vi "IBM4_Rate.vi"(8 "error in":errorcluster, 10 "Rate":i32=10000, 11 "COM resource in":refnum<visa-resource-name>="COM8") -> (0 "error out":errorcluster, 3 "COM resource out":refnum<visa-resource-name>="COM8")   [LabVIEW 2022 SP3, in "IBM4.lvlib"]
doc: "This VI interfaces with the IBM4 to perform a write operation where a Voltage is output on one of the analogue output pins of the IBM4.\n\nThe output channel must be 0 or 1, while the output value should be specified in Volts (thus, floating point)"
uses:
  <instrlib>/IBM4/IBM4.lvlib
panel:
  out "read buffer":string="Rate =  10000 SPS\r\n"
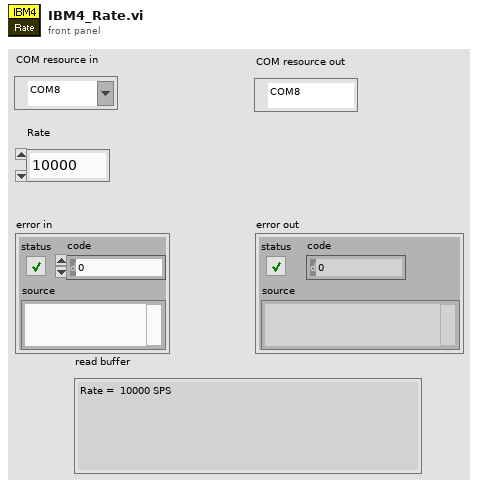
[diagram p1: front panel]
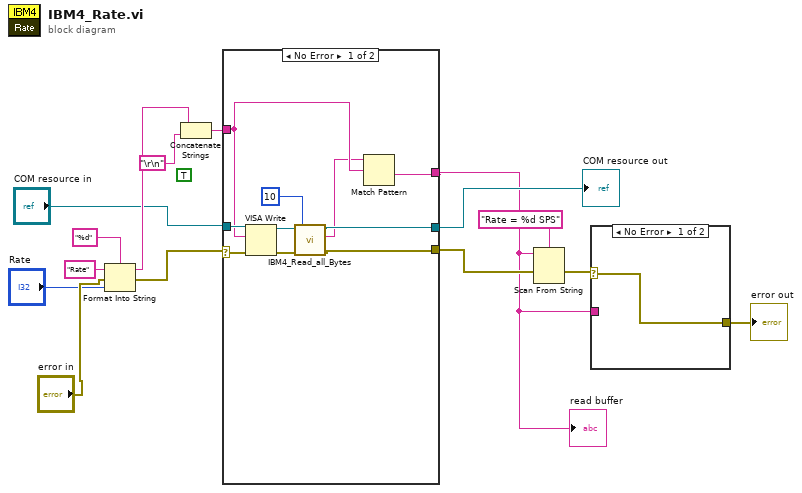
[diagram p0: block diagram]
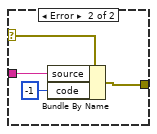
[diagram p2: hidden frame]
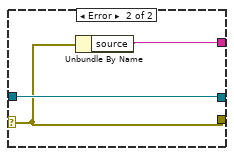
[diagram p3: hidden frame]
diagram:
  (unwired) TRUE ("Enable Termination\nChar (T)")
  n1 = Format Into String(format string="%d", initial string="Rate", error in="error in", "Rate") -> (resulting string=w7:string, error out=w1:errorcluster)
  n2 = Concatenate Strings(w7, "\r\n") -> (w6:string)
  n3 = case shown="No Error" w1 {
    selector: w1 -> [w22 w26]
    tunnel: "COM resource in" -> [w25 w28]
    tunnel: [w17 w26] -> w10
    tunnel: [w24 w27] -> w3
    tunnel: w6 -> [w23 _]
    tunnel: [w18 w28] -> w11
    frame No Error {
      n4 = VISA Write(VISA resource name=w25, write buffer=w23, error in (no error)=w22) -> (VISA resource name out=w21:refnum<visa-resource-name>, error out=w20:errorcluster)  [unwired: 1 out]
      n5 = call <instrlib>:"IBM4_Read_all_Bytes.vi"("error in (no error)"=w20, "milliseconds to wait"=u32 10, "VISA Refnum in"=w21) -> ("error out"=w17:errorcluster, "String"=w16:string, "VISA Refnum out"=w18:refnum<visa-resource-name>)  [unwired: 2 in]
      n6 = Match Pattern(string=w16, regular expression=w23) -> (after substring=w24:string)  [unwired: 1 in, 3 out]
    }
    frame Error {
      n7 = Unbundle By Name(w26) -> ("source"=w27:string)
    }
  }
  "COM resource out" <- w11
  "read buffer" <- w3
  n8 = Scan From String(format string="Rate = %d SPS", input string=w3, error in=w10) -> (error out=w5:errorcluster)  [unwired: 3 in, 2 out]
  n9 = case shown="No Error" w5 {
    selector: w5 -> [w29 w33]
    tunnel: [w29 w31] -> w4
    tunnel: w3 -> [_ w32]
    frame No Error {
    }
    frame Error {
      n10 = Bundle By Name(cluster=w33, "source"=w32, "code"=-1) -> (w31:errorcluster)
    }
  }
  "error out" <- w4
